vi "Test Assert Not Error Code.vi"(8 "error in (no error)":errorcluster) -> (0 "error out":errorcluster)   [LabVIEW 2013]
uses:
  classes/Assert/Assert.lvclass
  classes/Test/Test.lvclass
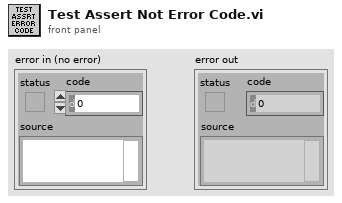
[diagram p1: front panel]
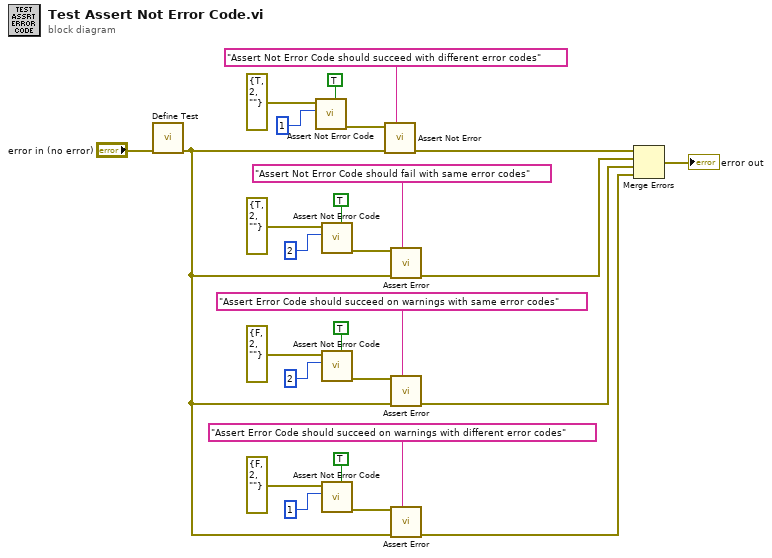
[diagram p0: block diagram]
diagram:
  n1 = call "Define Test.vi"("error in (no error)"="error in (no error)") -> ("error out"=w2:errorcluster)  [unwired: 9 in, 1 out]
  n2 = call "Assert Not Error Code.vi"("Assert Only? (F)"=TRUE, "Error Code"=1, "Error?"=errorcluster {"status"=TRUE, "code"=2, "source"=""}) -> ("error out"=w27:errorcluster)  [unwired: 7 in, 1 out]
  n3 = call "Assert Not Error Code.vi"("Assert Only? (F)"=TRUE, "Error Code"=2, "Error?"=errorcluster {"status"=TRUE, "code"=2, "source"=""}) -> ("error out"=w25:errorcluster)  [unwired: 7 in, 1 out]
  n4 = call "Assert Not Error Code.vi"("Assert Only? (F)"=TRUE, "Error Code"=2, "Error?"=errorcluster {"status"=FALSE, "code"=2, "source"=""}) -> ("error out"=w9:errorcluster)  [unwired: 7 in, 1 out]
  n5 = call "Assert Not Error Code.vi"("Assert Only? (F)"=TRUE, "Error Code"=1, "Error?"=errorcluster {"status"=FALSE, "code"=2, "source"=""}) -> ("error out"=w7:errorcluster)  [unwired: 7 in, 1 out]
  n6 = call "Assert Not Error.vi"("Label"="Assert Not Error Code should succeed with different error codes", "error in (no error)"=w2, "Not Error?"=w27) -> ("error out"=w19:errorcluster)  [unwired: 7 in, 1 out]
  n7 = call "Assert Error.vi"("Label"="Assert Not Error Code should fail with same error codes", "error in (no error)"=w2, "Error?"=w25) -> ("error out"=w20:errorcluster)  [unwired: 7 in, 1 out]
  n8 = call "Assert Error.vi"("Label"="Assert Error Code should succeed on warnings with same error codes", "error in (no error)"=w2, "Error?"=w9) -> ("error out"=w8:errorcluster)  [unwired: 7 in, 1 out]
  n9 = call "Assert Error.vi"("Label"="Assert Error Code should succeed on warnings with different error codes", "error in (no error)"=w2, "Error?"=w7) -> ("error out"=w1:errorcluster)  [unwired: 7 in, 1 out]
  n10 = Merge Errors(w19, w20, w8, w1) -> (→"error out":errorcluster)
